vi "Read Color Cluster.vi"(8 "error in (no error)":errorcluster, 9 "Active Plot":i32, 11 "3D Surface in":refnum<class "3D Surface.lvclass">) -> (0 "error out":errorcluster, 2 "Color Ramp Cluster":T1={"Color Ramp Style"=enum."None", "Color Ramp Array"=[16711934, 393471, 57855, 4390754, 16449346, 16744722, 16711680], "Color Ramp Index"=[45, 91, 133, 175, 219, 255], "Interpolate?"=FALSE, "Logarithm?"=FALSE}, 3 "3D Surface out":refnum<class "3D Surface.lvclass">)   [LabVIEW 2020, in "3D Surface.lvclass"]
uses:
  <vilib>/Math Plots/3D Math Plots/3D Surface/3D Surface/3D Surface.lvclass
  <vilib>/Math Plots/3D Math Plots/3D Plot/3D Plot/Typedef/Color Ramp Cluster.ctl
  <vilib>/Math Plots/3D Math Plots/3D Surface/3D Surface/3D Surface.lvclass/3D Surface.ctl
  <vilib>/Math Plots/3D Math Plots/3D Plot/3D Plot/3D Plot.lvclass
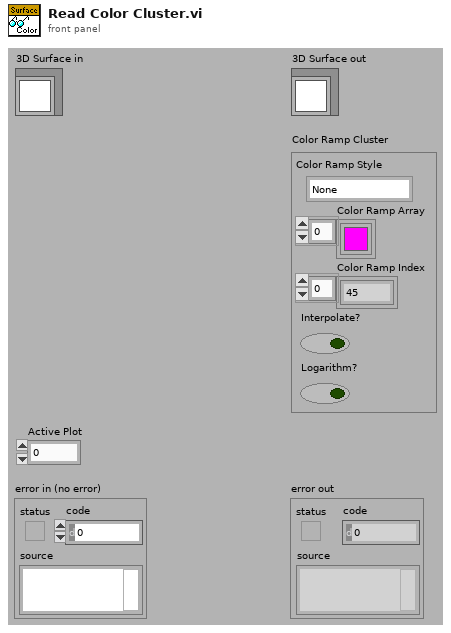
[diagram p1: front panel]
types:
  T1 = typedef "3D Plot.lvclass/Color Ramp Cluster.ctl" = cluster{"Color Ramp Style":enum16{"None", "Shaded", "Color spectrum", "Grey scale", "Custom"}, "Color Ramp Array":u32[], "Color Ramp Index":i32[], "Interpolate?":bool, "Logarithm?":bool}
  T2 = typedef "3D Surface.lvclass/3D Surface Property Array.ctl" = T3[]
  T3 = typedef "3D Surface.lvclass/3D Surface Property.ctl" = cluster{"General Property":cluster{"Plot Name":string, "Coordinate System":enum16{"Cartesian", "Cylindrical", "Spherical"}, "Opacity":sgl}, "Projection Property":cluster{"Draw XY":bool, "Draw YZ":bool, "Draw XZ":bool}, "Plot Property":cluster{"Draw Surface":bool, "Draw Mesh":bool, "Draw Normal":bool, "Color Ramp Cluster":T1, "Line Style":T4, "Line Width":sgl, "Line Color":u32, "Antialiasing":bool}, "Surface Property":cluster{"Color Mode":enum16{"Flat Shading", "Interpolated Shading"}}}
  T4 = typedef "3D Plot.lvclass/Line Type.ctl" = enum16{"None", "Solid", "Dash", "Dot", "Dash Dot"}
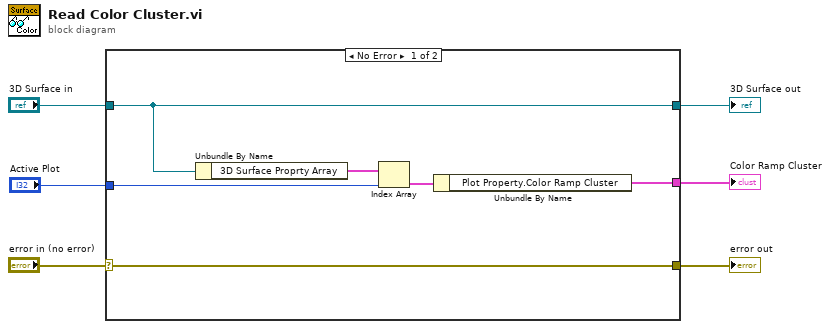
[diagram p0: block diagram]
diagram:
  n1 = case shown="No Error" "error in (no error)" {
    selector: "error in (no error)" -> [w12 w14]
    tunnel: [w12 w14] -> w2
    tunnel: [w11 _] -> w3
    tunnel: "3D Surface in" -> [w10 w13]
    tunnel: [w10 w13] -> w5
    tunnel: "Active Plot" -> [w9 _]
    frame No Error {
      n2 = Unbundle By Name(w10) -> ("3D Surface Proprty Array"=w8:T2)
      n3 = Index Array(array=w8, index=w9) -> (element=w7:T3)
      n4 = Unbundle By Name(w7) -> ("Plot Property.Color Ramp Cluster"=w11:T1)
    }
    frame Error {
    }
  }
  "error out" <- w2
  "3D Surface out" <- w5
  "Color Ramp Cluster" <- w3
